vi "Analyze Data.vi"(8 "error in":errorcluster, 11 "PAS in":refnum<class "PAS.lvclass">) -> (0 "error out":errorcluster, 3 "PAS out":refnum<class "PAS.lvclass">)   [LabVIEW 2014, in "PAS Library.lvlib" / "PAS.lvclass"]
doc: "This is the core routine for PAS microphone data analysis. Here, the microphone data is retrieved from each of the cells. In both cases, the time domain signal will be transformed to the frequency domain. If the speaker is on (<B>Spk Pos</B> == TRUE), then the frequency domain signal will be squared to obtain the power and a Lorentzian will be fit to the data to retrieve the resonant characteristics of the cell. If the speaker is off (<B>Spk Pos</B> == FALSE), then the amplitude will be used to calculate the integrated area of the signal. In every case, the implementation has the ability to decimate the data for transmission of the waveforms over a network line."
uses:
  PAS.lvclass
  Data/Main/PAS Data.lvclass
  PAS.lvclass/PAS.ctl
  Instrument/Instrument.lvclass/Instrument.ctl
  <vilib>/Analysis/4window.llb/windowTd.ctl
  Instrument/Read Data.vi
  Instrument/Write Data.vi
  Read Chirp.vi
  Get Speaker State.vi
  Read Cells.vi
  Data/Main/Write drive.vi
  Data/Main/Read CellData.vi
  Data/Main/Read filter.vi
  Cell/Read extParams.vi
  <vilib>/measure/maspectr.llb/FFT Spectrum (Mag-Phase) for 1 Chan.vi
  Data/Cell/Get Integrated Area.vi
  Write Cells.vi
  Data/Data.lvlibp/Data.lvclass
  Cell/PAS Cell.lvclass
  Data/Cell/PAS Cell Data.lvclass
  <vilib>/Analysis/NI_AALPro.lvlib
  Instrument/Instrument.lvclass
  <vilib>/measure/NI_MAPro.lvlib
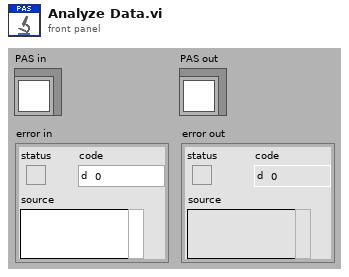
[diagram p1: front panel]
types:
  T1 = typedef "NI_AALPro.lvlib/windowTd.ctl" = u32
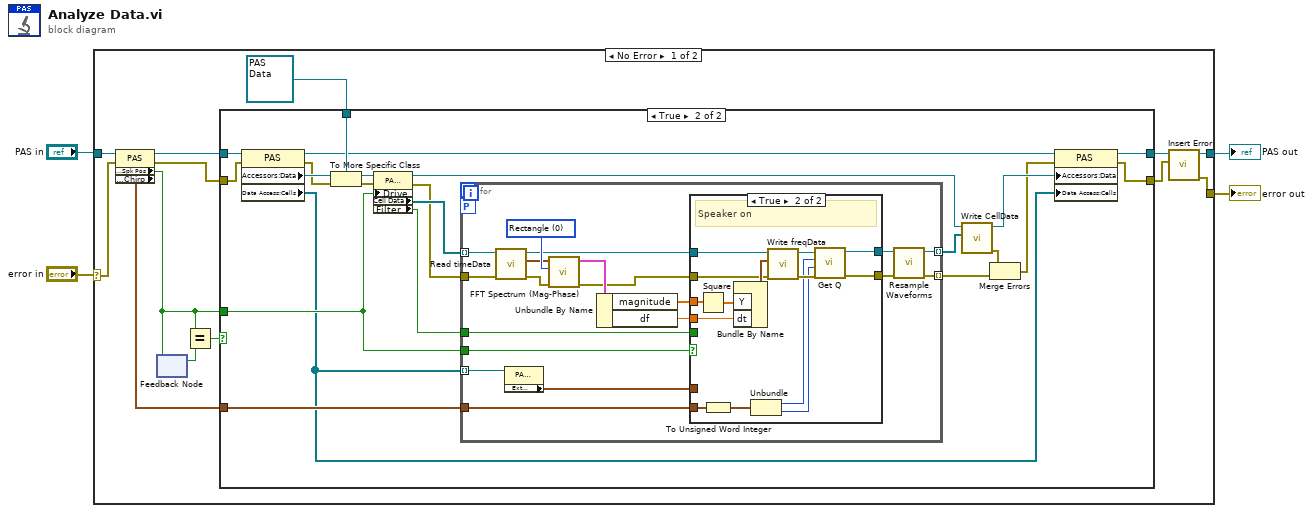
[diagram p0: block diagram]
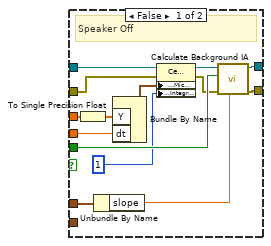
[diagram p3: hidden frame]
diagram:
  n1 = case shown="No Error" "error in" {
    selector: "error in" -> [w11 w90]
    tunnel: [w15 w90] -> w1
    tunnel: [w16 w89] -> w2
    tunnel: "PAS in" -> [w14 w89]
    frame No Error {
      n2 = property class="PAS"(reference=w14, error in=w11) -> (reference out=w13:refnum<class "PAS.lvclass">, error out=w12:errorcluster, "Data Access:Spk Pos"=w6:bool, "Data Access:Chirp"=w10:cluster{"f_center":dbl, "bandwidth":dbl})
      n3 = feedback-in #1(w6) -> ()
      n4 = feedback #1() -> (w7:bool)  [unwired: 1 in]
      n5 = Equal?(x=w6, y=w7) -> (x = y?=w8:bool)
      n6 = case shown="True" w8 {
        tunnel: [w19 w24] -> w17
        tunnel: w13 -> [w19 w38]
        tunnel: w12 -> [w18 w23]
        tunnel: w6 -> [_ w41]
        tunnel: w10 -> [_ w40]
        tunnel: [w18 w20] -> w9
        tunnel: refnum<class "PAS Data.lvclass"> refnum ("reference") -> [_ w39]
        frame False {
        }
        frame True {
          n7 = property class="PAS"(reference=w38, error in=w23) -> (reference out=w26:refnum<class "PAS.lvclass">, error out=w22:errorcluster, "Accessors:Data"=w28:refnum<class "Data.lvclass">, "Data Access:Cells"=w25:refnum<class "PAS Cell.lvclass">[])
          n8 = To More Specific Class(target class=w39, reference=w28, error in=w22) -> (specific class reference=w30:refnum<class "PAS Data.lvclass">, error out=w29:errorcluster)
          n9 = property class="PAS Data"(reference=w30, error in=w29, "Drive"=w41) -> (reference out=w33:refnum<class "PAS Data.lvclass">, error out=w32:errorcluster, "Cell Data"=w34:refnum<class "PAS Cell Data.lvclass">[], "Filter"=w31:bool)
          n10 = for {
            tunnel: w34 -> [w60] mode=indexing
            tunnel: [w57] -> w37 mode=indexing
            tunnel: [w56] -> w36 mode=indexing
            workers-P: _ -> [_]
            tunnel: w41 -> [w46]
            tunnel: w32 -> [w47]
            tunnel: w25 -> [w45] mode=indexing
            tunnel: w40 -> [w43]
            tunnel: w31 -> [w42]
            w55 = T1 0 items=["Rectangle"=0, "Hanning"=1, "Hamming"=2, "Blackman-Harris"=3, "Exact Blackman"=4, "Blackman"=5, "Flat Top"=6, "4 Term B-Harris "=7, "7 Term B-Harris"=8, "Low Sidelobe"=9, "Blackman Nuttall"=11, "Triangle"=30, "Bartlett-Hanning"=31, "Bohman"=32, "Parzen"=33, "Welch"=34, "Kaiser"=60, "Dolph-Chebyshev"=61, "Gaussian"=62] ("window")
            n11 = call "Read timeData.vi"("error in"=w47, "PAS Cell Data in"=w60) -> ("error out"=w53:errorcluster, "timeData"=w52:waveform(i16), "PAS Cell Data out"=w50:refnum<class "PAS Cell Data.lvclass">)  [unwired: 7 in]
            n12 = property class="PAS Cell"(reference=w45) -> ("Ext Params"=w44:cluster{"slope":sgl, "zero":sgl})  [unwired: 1 in, 2 out]
            n13 = call-poly <vilib>:"FFT Spectrum (Mag-Phase).vi"("error in (no error)"=w53, "window"=w55, "time signal"=w52) -> ("error out"=w51:errorcluster, "magnitude"=w54:cluster{"f0":dbl, "df":dbl, "magnitude":dbl[]})  [unwired: 4 in, 3 out]
            n14 = Unbundle By Name(w54) -> ("magnitude"=w49:dbl[], "df"=w48:dbl)
            n15 = case shown="True" w46 {
              tunnel: w50 -> [w66 w82]
              tunnel: w51 -> [w63 w81]
              tunnel: [w72 w88] -> w58
              tunnel: [w73 w87] -> w59
              tunnel: w49 -> [w68 w80]
              tunnel: w48 -> [w74 w84]
              tunnel: w44 -> [w70 _]
              tunnel: w43 -> [_ w76]
              tunnel: w42 -> [w71 _]
              frame False {
                # "Speaker Off"
                n16 = To Single Precision Float(number=w68) -> (single precision float=w67:sgl[])
                n17 = Unbundle By Name(w70) -> ("slope"=w69:sgl)
                n18 = Bundle By Name("Y"=w67, "dt"=w74) -> (w64:waveform(sgl))  [unwired: 1 out]
                n19 = property class="Cell Data"(reference=w66, error in=w63, "Accessors:Mic Frequency"=w64, "Accessors:Integrated Area"=1 ("Integrated Area")) -> (reference out=w61:refnum<class "PAS Cell Data.lvclass">, error out=w62:errorcluster)
                n20 = call "Calculate Background IA.vi"("Slope"=w69, "error in"=w62, "Filter"=w71, "Cell Data in"=w61) -> ("error out"=w72:errorcluster, "Cell Data out"=w73:refnum<class "PAS Cell Data.lvclass">)  [unwired: 6 in]
              }
              frame True {
                # "Speaker on"
                n21 = Square(x=w80) -> (x^2=w79:dbl[])
                n22 = To Unsigned Word Integer(number=w76) -> (unsigned 16bit integer=w75:cluster{"f_center":u16, "bandwidth":u16})
                n23 = Bundle By Name("Y"=w79, "dt"=w84) -> (w83:waveform(dbl))  [unwired: 1 out]
                n24 = Unbundle(w75) -> ("f_center"=w78:u16, "bandwidth"=w77:u16)
                n25 = call "Write freqData.vi"("error in (no error)"=w81, "freqData"=w83, "PAS Cell Data in"=w82) -> ("error out"=w85:errorcluster, "PAS Cell Data out"=w86:refnum<class "PAS Cell Data.lvclass">)  [unwired: 7 in]
                n26 = call "Get Q.vi"("error in"=w85, "Bandwidth"=w77, "f_center"=w78, "PAS Cell Data in"=w86) -> ("error out"=w88:errorcluster, "PAS Cell Data out"=w87:refnum<class "PAS Cell Data.lvclass">)  [unwired: 6 in]
              }
            }
            n27 = call "Resample Waveforms.vi"("error in"=w58, "PAS Cell Data in"=w59) -> ("error out"=w56:errorcluster, "PAS Cell Data out"=w57:refnum<class "PAS Cell Data.lvclass">)  [unwired: 8 in]
          }
          n28 = call "Write CellData.vi"("CellData"=w37, "PAS Data in"=w33) -> ("error out"=w35:errorcluster, "PAS Data out"=w27:refnum<class "PAS Data.lvclass">)  [unwired: 8 in]
          n29 = Merge Errors(w35, w36) -> (w21:errorcluster)
          n30 = property class="PAS"(reference=w26, error in=w21, "Accessors:Data"=w27, "Data Access:Cells"=w25) -> (reference out=w24:refnum<class "PAS.lvclass">, error out=w20:errorcluster)
        }
      }
      n31 = call "Insert Error.vi"("err"=w9, "Instrument in"=w17) -> ("error out"=w15:errorcluster, "Instrument out"=w16:refnum<class "PAS.lvclass">)  [unwired: 7 in, 1 out]
    }
    frame Error {
    }
  }
  "error out" <- w1
  "PAS out" <- w2
